vi "zeropatch.vi"   [LabVIEW 2015]
uses:
  <vilib>/DAQmx/write.llb/DAQmx Write (Analog DBL 1Chan 1Samp).vi
  <vilib>/DAQmx/create/channels.llb/DAQmx Create Channel (AO-Voltage-Basic).vi
  <vilib>/DAQmx/miscellaneous.llb/DAQmx Fill In Error Info.vi
types:
  T1 = typedef "XYZStage.lvlib/XYZStage Configuration.ctl" = cluster{"VISA resource name":refnum<visa-resource-name>, "Timeout (3sec)":u32}
  T2 = cluster{"StageS":i32, "StageL":i32, "currmeas data dir":path, "image OD":u16, "contour OD":u16, "point OD":u16, "AOlines":tag[], "AIlines":tag[], "CI lines":tag[], "DO lines":tag[], "AO names":string[], "CI names":string[], "AI names":string[], "DO names":string[], "CIextensions":string[], "AIextensions":string[], "Voltage to Ygalvo":i32, "Voltage to Xgalvo":i32, "Voltage to patch":i32, "640 shutter":i32, "2P shutter":i32, "LT timestamp":u32, "Vp":i32, "Ip":i32, "camera trigger":i32, "master data dir":path, "voltage to Zpos":i32, "Vto2P":i32, "640 AO":i32, "488 AO":i32, "532 AO":i32, "640TTL":u32, "488TTL":u32, "532TTL":u32, "Device 1 sampleclock out":tag, "Device 1 Starttrigger out":tag, "Device 2 sampleclock in":tag, "Device 2 StartTrigger in ":tag, "2PODTTL":u32, "488 shutter":u32, "LCVR red":u32, "LCVR blue":u32, "Sutter Stage Config":T1, "Device 1 ext sampleclock in (100Khz)":tag}
  T3 = cluster{"VC":bool, "CC":bool, "CC_icg (pA/mv)":sgl, "VC_icg (mV/mV)":sgl, "OCG (mV/pA)":sgl, "OVG (mV/mV)":dbl, "Vhold (mV)":sgl, "holdon":bool}
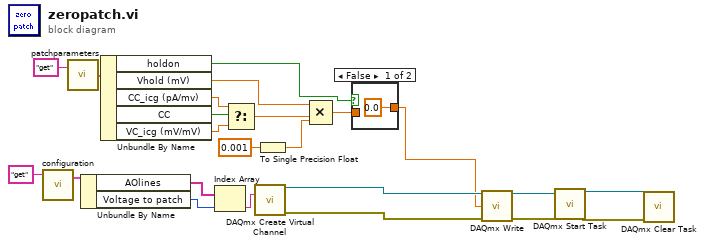
[diagram p0: block diagram]
diagram:
  n1 = call "configuration.vi"("command"="get") -> ("config out"=w22:T2)  [unwired: 2 in, 1 out]
  n2 = call "patchparameters.vi"("command"="get") -> ("Params out"=w15:T3)  [unwired: 1 in]
  n3 = Unbundle By Name(w22) -> ("AOlines"=w5:tag[], "Voltage to patch"=w4:i32)
  n4 = Unbundle By Name(w15) -> ("holdon"=w16:bool, "Vhold (mV)"=w17:sgl, "CC_icg (pA/mv)"=w9:sgl, "CC"=w11:bool, "VC_icg (mV/mV)"=w10:sgl)
  n5 = Index Array(array=w5, index=w4) -> (element=w3:tag)
  n6 = Select(t=w9, s=w11, f=w10) -> (s? t:f=w8:sgl)
  n7 = call-poly <vilib>:"DAQmx Create Virtual Channel.vi"("physical channels"=w3) -> ("task out"=w20:refnum<k21>, "error out"=w21:errorcluster)  [unwired: 13 in]
  n8 = To Single Precision Float(number=0.001 ("y")) -> (single precision float=w7:sgl)
  n9 = Compound Arithmetic op=MULTIPLY(w17, w8, w7) -> (w13:sgl)
  n10 = case shown="False" w16 {
    tunnel: w13 -> [_ w25]
    tunnel: [0.0 w25] -> w6
    frame False {
    }
    frame True {
    }
  }
  n11 = call-poly <vilib>:"DAQmx Write.vi"("task/channels in"=w20, "data"=w6, "error in"=w21) -> ("task out"=w19:refnum<k21>, "error out"=w18:errorcluster)  [unwired: 10 in, 1 out]
  n12 = call <vilib>:"DAQmx Start Task.vi"("task/channels in"=w19, "error in"=w18) -> ("task out"=w2:refnum<k21>, "error out"=w1:errorcluster)  [unwired: 12 in]
  n13 = call <vilib>:"DAQmx Clear Task.vi"("task in"=w2, "error in"=w1) -> ()  [unwired: 13 in, 1 out]
